vi "test.vi"() -> ()   [LabVIEW 2019]
panel:
  in  "duration":dbl
  in  "start":dbl
  in  "peak":dbl
  out "XY Graph":cluster{"Array":dbl[], "torques":dbl[]}(graph)
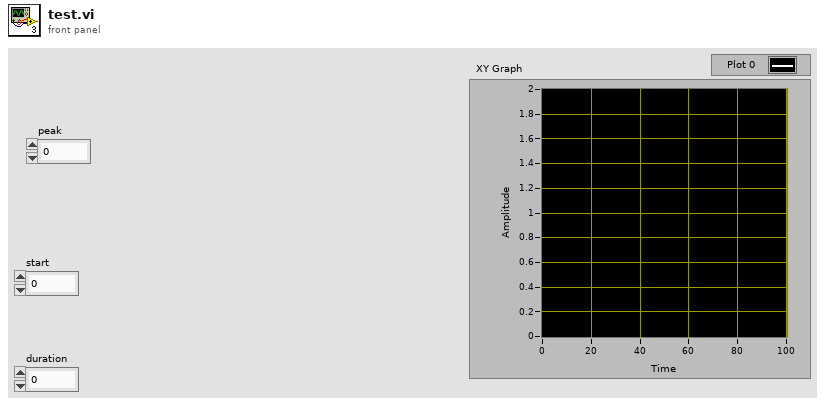
[diagram p1: front panel]
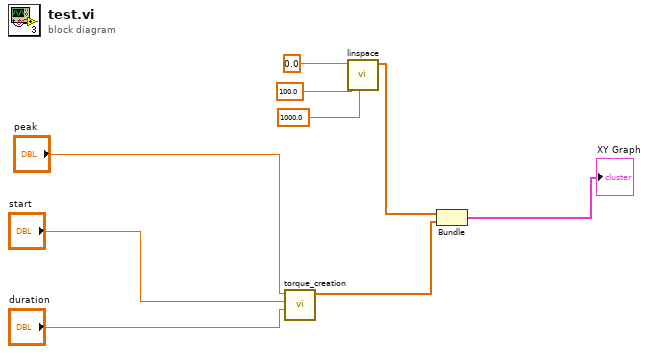
[diagram p0: block diagram]
diagram:
  n1 = call "torque_creation.vi"("duration"="duration", "start"="start", "peak"="peak") -> ("torques"=w2:dbl[])  [unwired: 8 in]
  n2 = call "linspace.vi"("NumElements"=1000.0, "End"=100.0, "Start"=0.0) -> ("Array"=w3:dbl[])  [unwired: 8 in]
  n3 = Bundle("Array"=w3, "torques"=w2) -> (→"XY Graph":cluster{"Array":dbl[], "torques":dbl[]})  [unwired: 1 in]
